vi "Test FTP.vi"() -> ()   [LabVIEW 2012]
uses:
  <vilib>/FTP/ftp2.llb/FTP File Info.ctl
  <vilib>/FTP/NI_FTP.lvlib
panel:
  out "reply code 2":i32
  out "dir list":T1[](array[typedef])
  out "error out 3":errorcluster
  out "reply code":i32
  out "data":string
  out "file error":errorcluster
  out "error out":errorcluster
  in  "host":string
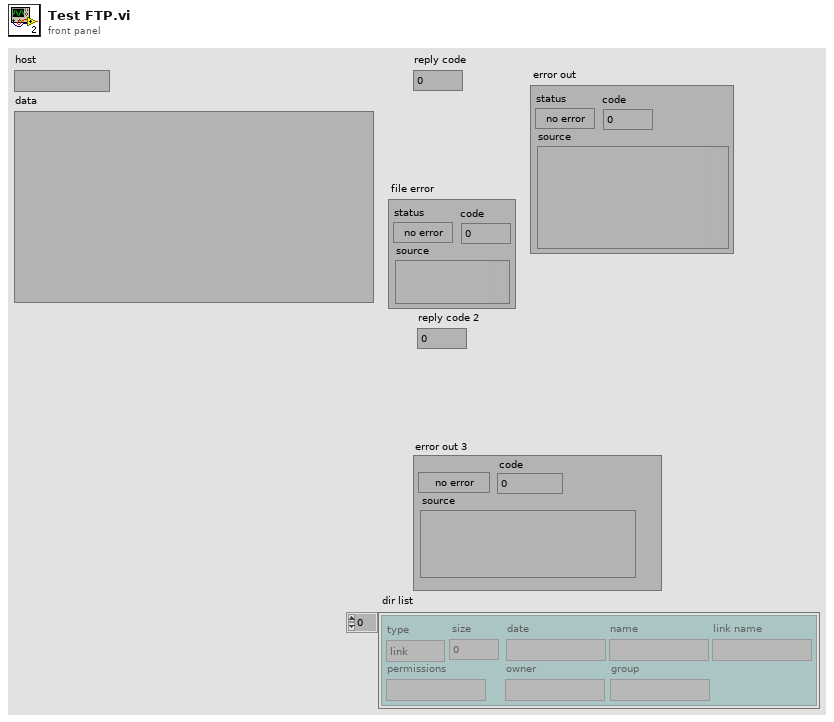
[diagram p1: front panel]
types:
  T1 = typedef "NI_FTP.lvlib/FTP File Info.ctl" = cluster{"type":enum16{"unknown", "file", "dir", "link"}, "permissions":string, "owner":string, "group":string, "size":i32, "date":string, "name":string, "link name":string}
  T2 = typedef "NI_FTP.lvlib/FTP Session.ctl" = refnum<k5>
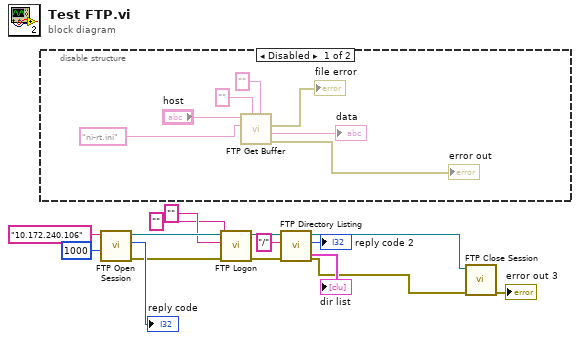
[diagram p0: block diagram]
diagram:
  n1 = disable-structure shown="Disabled" {
    frame Disabled {
      n2 = call <vilib>:"FTP Get Buffer.vi"("password"="", "user"="", "remote path"="ni-rt.ini", "host"="host") -> ("error out"=→"error out":errorcluster, "data"=→"data":string, "file error"=→"file error":errorcluster)  [unwired: 5 in]
    }
    frame Enabled {
    }
  }
  n3 = call <vilib>:"FTP Open Session.vi"("timeout ms (60000)"=1000, "address"="10.172.240.106") -> ("error out"=w10:errorcluster, "reply code"=→"reply code":i32, "ftp session"=w11:T2)  [unwired: 6 in, 1 out]
  n4 = call <vilib>:"FTP Logon.vi"("error in (no error)"=w10, "password"="", "user"="", "ftp session"=w11) -> ("error out"=w6:errorcluster, "ftp session out"=w7:T2)  [unwired: 4 in, 2 out]
  n5 = call <vilib>:"FTP Directory Listing.vi"("error in (no error)"=w6, "directory path"="/", "ftp session"=w7) -> ("error out"=w4:errorcluster, "reply code"=→"reply code 2":i32, "ftp session out"=w3:T2, "dir list"=→"dir list":T1[])  [unwired: 4 in, 1 out]
  n6 = call <vilib>:"FTP Close Session.vi"("error in (no error)"=w4, "ftp session"=w3) -> ("error out"=→"error out 3":errorcluster)  [unwired: 6 in, 3 out]
